vi "Actor Setup.vi"(10 "Actor":refnum<class "Actor.lvclass">, 11 "Actor in":refnum<class "Self Actor.lvclass">) -> (0 "error out":errorcluster, 3 "Actor out":refnum<class "Self Actor.lvclass">)   [LabVIEW 2021, in "LVCAM.lvlib" / "Self Actor.lvclass"]
uses:
  Self Actor.lvclass
  Actor/Actor.lvclass
  Self Actor.lvclass/Self Actor.ctl
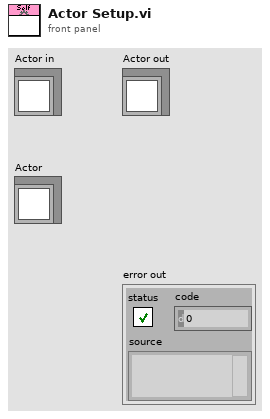
[diagram p1: front panel]
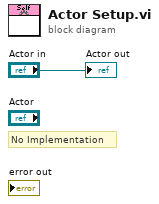
[diagram p0: block diagram]
diagram:
  # "No Implementation"
  "Actor out" <- "Actor in"
